vi "Read Voltage.vi"(8 "error in (no error)":errorcluster, 11 "Set Output Voltage Msg in":refnum<class "Set Output Voltage Msg.lvclass">) -> (0 "error out":errorcluster, 2 "Voltage":dbl[unit], 3 "Set Output Voltage Msg out":refnum<class "Set Output Voltage Msg.lvclass">)   [LabVIEW 2016, in "BNT_DAQmx.lvlib" / "Set Output Voltage Msg.lvclass"]
uses:
  Set Output Voltage Msg.lvclass
  Set Output Voltage Msg.lvclass/Set Output Voltage Msg.ctl
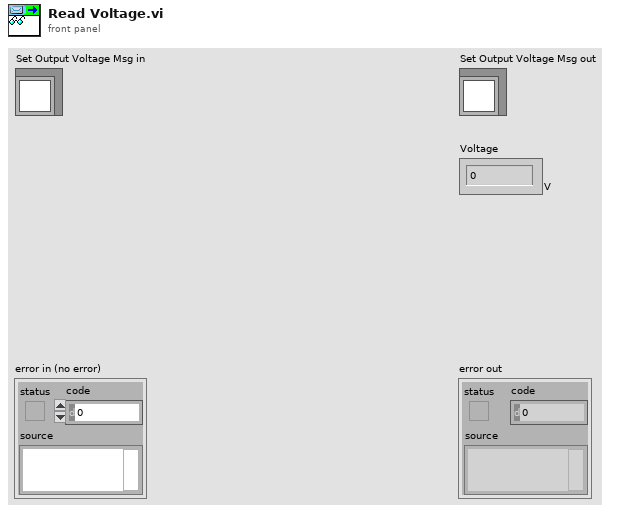
[diagram p1: front panel]
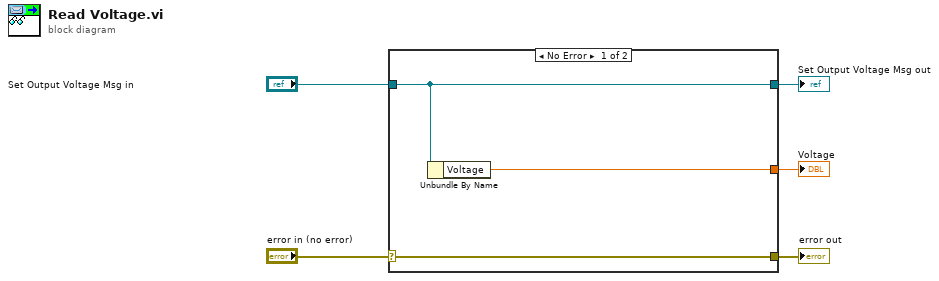
[diagram p0: block diagram]
diagram:
  n1 = case shown="No Error" "error in (no error)" {
    selector: "error in (no error)" -> [w8 w9]
    tunnel: [w8 w9] -> w4
    tunnel: [w7 w10] -> w2
    tunnel: "Set Output Voltage Msg in" -> [w7 w10]
    tunnel: [w6 _] -> w1
    frame No Error {
      n2 = Unbundle By Name(w7) -> ("Voltage"=w6:dbl[unit])
    }
    frame Error {
    }
  }
  "error out" <- w4
  "Set Output Voltage Msg out" <- w2
  "Voltage" <- w1
